vi "Run.vi"(8 "error in (no error)":errorcluster, 11 "Run in":refnum<class "LUnit Test Suite V2.lvclass">) -> (0 "error out":errorcluster, 2 "Results":T1[](array[typedef]))   [LabVIEW 2020, in "LUnit Test Suite V2.lvclass"]
uses:
  LUnit Test Suite V2.lvclass
  Result/Result.ctl
  Result/Status.ctl
  Result/Type.ctl
  LUnit Test Suite V2.lvclass/LUnit Test Suite V2.ctl
  Run/Runnable.lvclass
  Result/Result.lvlib
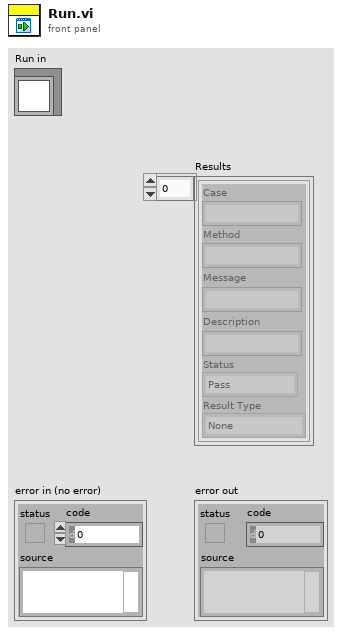
[diagram p1: front panel]
types:
  T1 = typedef "Result.lvlib/Result.ctl" = cluster{"Case":string, "Method":string, "Message":string, "Description":string, "Status":T2, "Result Type":T3}
  T2 = typedef "Result.lvlib/Status.ctl" = enum16{"Pass", "Fail", "Error", "Skipped", "Setup Error", "Broken", "Teardown Error"}
  T3 = typedef "Result.lvlib/Type.ctl" = enum16{"None", "Pass", "Fail", "Skip", "Pass if Equal", "Fail if Equal", "Pass if Error", "Fail if Error", "Pass if", "Fail if"}
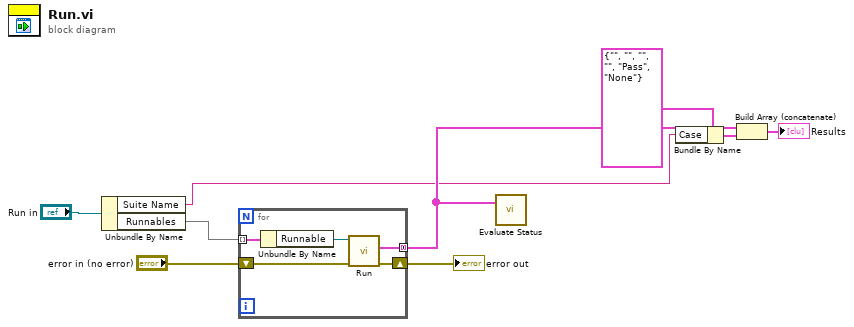
[diagram p0: block diagram]
diagram:
  n1 = Unbundle By Name("Run in") -> ("Suite Name"=w1:string, "Runnables"=w8:map{string, refnum<class "Runnable.lvclass">})
  n2 = for {
    tunnel: w8 -> [w14] mode=indexing
    shift-right: [w12] -> w6
    shift-left: "error in (no error)" -> [w13]
    tunnel: [w11] -> w5 mode=concatenating
    n3 = Unbundle By Name(w14) -> ("Runnable"=w10:refnum<class "Runnable.lvclass">)
    n4 = call-dynamic "Run.vi"("error in (no error)"=w13, "Run in"=w10) -> ("error out"=w12:errorcluster, "Results"=w11:T1[])  [unwired: 8 in]
  }
  "error out" <- w6
  n5 = call "Evaluate Status.vi"("Results"=w5) -> ()  [unwired: 10 in, 1 out]
  n6 = Bundle By Name(cluster=T1 {"Case"="", "Method"="", "Message"="", "Description"="", "Status"=enum."Pass", "Result Type"=enum."None"} ("Results"), "Case"=w1) -> (w2:T1)
  n7 = Build Array (concatenate)(w5, w2) -> (→"Results":T1[])
